vi "csi to u64.vi"(11 "subcarrier channel":T1) -> (3 "Numeric":u64)   [LabVIEW 2020]
types:
  T1 = cluster{"Real":fxp<+/-,25,4>, "Imag":fxp<+/-,25,4>}
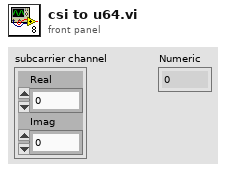
[diagram p1: front panel]
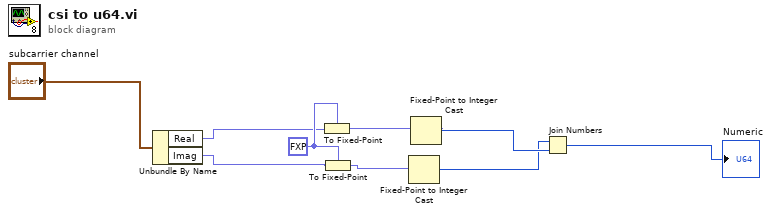
[diagram p0: block diagram]
diagram:
  w5 = fxp<+/-,32,11> 0.0 ("fixed-point type")
  n1 = Unbundle By Name("subcarrier channel") -> ("Real"=w3:fxp<+/-,25,4>, "Imag"=w4:fxp<+/-,25,4>)
  n2 = To Fixed-Point(fixed-point type=w5, number=w3) -> (fixed-point=w6:fxp<+/-,32,11>)
  n3 = To Fixed-Point(fixed-point type=w5, number=w4) -> (fixed-point=w7:fxp<+/-,32,11>)
  n4 = Fixed-Point to Integer Cast(1:w7) -> (0:w8:i32)
  n5 = Fixed-Point to Integer Cast(1:w6) -> (0:w9:i32)
  n6 = Join Numbers(hi=w8, lo=w9) -> ((hi.lo)=→"Numeric":u64)
